vi "Request Audio Summary.vi"(11 "VMR Actor API in":refnum<class "VMR Actor API.lvclass">) -> (0 "error out":errorcluster, 2 "Audio Summary":T1)   [LabVIEW 2022 SP3, in "VMR Server.lvlib" / "VMR Actor API.lvclass"]
uses:
  VMR Actor API.lvclass
  VMR Actor API.lvclass/VMR Actor API.ctl
  VMR Actor Messages/Request Summary Msg/Request Summary Msg.lvclass
  <vilib>/IlluminatedG/IG Promises/Promises/Promise/Promise.lvclass
  AudioSummaryValue/AudioSummaryValue.lvclass
  C:/Program Files (x86)/National Instruments/LabVIEW 2022/vi.lib/IlluminatedG/IG Promises/Promises/Value/Value.lvclass
  C:/dev/lv/2022/touchcontrol/VMR Server/AudioSummaryValue/AudioSummaryValue.lvclass
  <vilib>/IlluminatedG/IG Promises/Promises/Future/Future.lvclass
  VMR Server Shared/Channel.ctl
  VMR Server Shared/VMR Server Shared.lvlib
  VMR Server Shared/Audio Summary.ctl
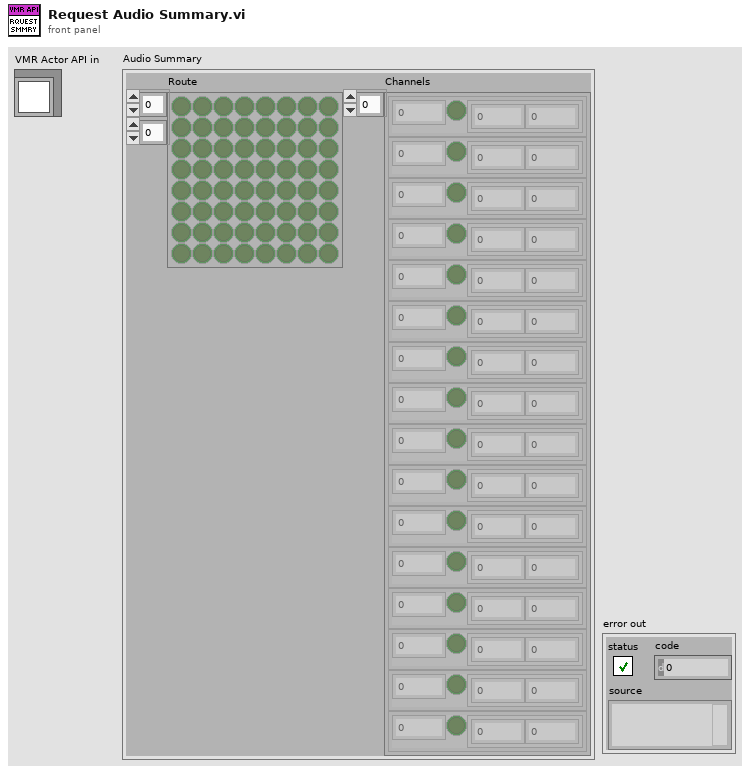
[diagram p1: front panel]
types:
  T1 = typedef "VMR Server Shared.lvlib/Audio Summary.ctl" = cluster{"Route":bool[][], "Channels":T2[]}
  T2 = typedef "VMR Server Shared.lvlib/Channel.ctl" = cluster{"Volume":dbl, "Muted":bool, "Levels":cluster{"L":dbl, "R":dbl}}
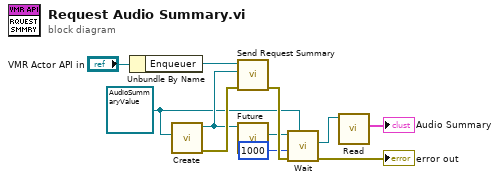
[diagram p0: block diagram]
diagram:
  w5 = refnum<class "AudioSummaryValue.lvclass"> refnum ("VMR Server.lvlib:AudioSummaryValue.lvclass")
  n1 = Unbundle By Name("VMR Actor API in") -> ("Enqueuer"=w8:refnum<class "Message Enqueuer.lvclass">)
  n2 = call <vilib>:"Create.vi"("Result Type"=w5) -> ("error out"=w10:errorcluster, "Promise"=w7:refnum<class "Promise.lvclass">)  [unwired: 9 in]
  n3 = call "Send Request Summary.vi"("error in (no error)"=w10, "Promise"=w7, "Message Enqueuer"=w8) -> ("error out"=w11:errorcluster)  [unwired: 7 in, 1 out]
  n4 = call <vilib>:"Future.vi"("Promise in"=w7) -> ("Future"=w6:refnum<class "Future.lvclass">)  [unwired: 9 in, 1 out]
  n5 = call <vilib>:"Wait.vi"("Result Type"=w5, "error in (no error)"=w11, "Timeout mS (-1)"=1000, "Future in"=w6) -> ("error out"=→"error out":errorcluster, "Result"=w2:refnum<class "AudioSummaryValue.lvclass">)  [unwired: 6 in]
  n6 = call "Read.vi"("AudioSummaryValue in"=w2) -> ("Audio Summary"=→"Audio Summary":T1)  [unwired: 10 in]
